vi "BotSpeak_GetVer.vi"(3 "Bot Settings":T1) -> (0 "version":string, 1 "Bot Settings out":T1)   [LabVIEW 2012]
doc: "Returns the version number of the device's VM"
uses:
  <userlib>/botspeak/VIs/Direct/BotSpeak_Control.ctl
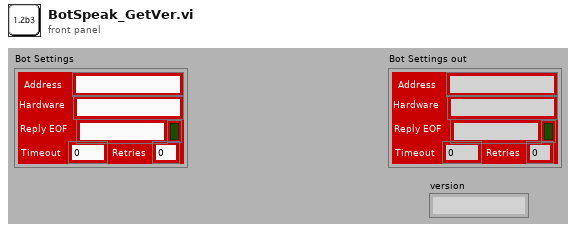
[diagram p1: front panel]
types:
  T1 = typedef "BotSpeak_Control.ctl" = cluster{"Address":string, "Reply EOF":string, "Hardware":string, "Retries":i8, "Timeout":i32, "Open?":bool}
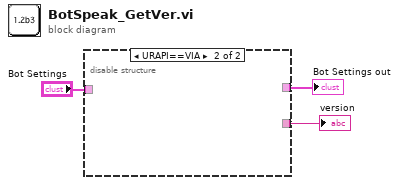
[diagram p0: block diagram]
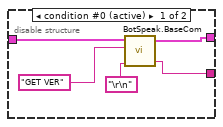
[diagram p2: hidden frame]
diagram:
  n1 = disable-structure shown="URAPI==VIA" {
    disable-tunnel: "Bot Settings" -> [w7 _]
    disable-tunnel: [w6 _] -> w2
    disable-tunnel: [w5 _] -> w1
    frame condition #0 (active) {
      n2 = call <userlib>:"BotSpeak.BaseCom.vi"("Termination"="\r\n", "command"="GET VER", "Bot Settings in"=w7) -> ("response"=w5:string, "Bot Settings out"=w6:T1)  [unwired: 2 in]
    }
    frame condition #1 {
    }
  }
  "version" <- w1
  "Bot Settings out" <- w2
